vi "Serial Log Driver.vi"(5 "Scanner 2?  (Scanner1)":bool, 7 "Valid Serial #":bool, 11 "error in (no error)":errorcluster, 12 "Write Text":string[](array[string]), 14 "operation":T1) -> (15 "error out":errorcluster)   [LabVIEW 2013]
uses:
  Controls/File Driver States.ctl
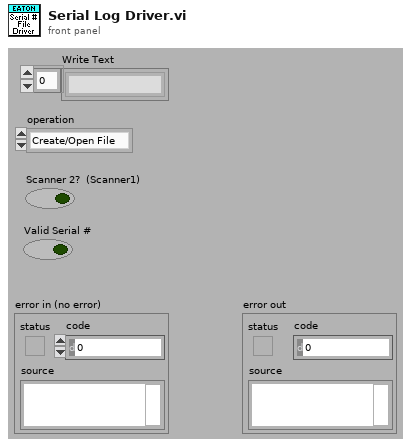
[diagram p1: front panel]
types:
  T1 = typedef "File Driver States.ctl" = enum16{"Create/Open File", "Write File", "Close File"}
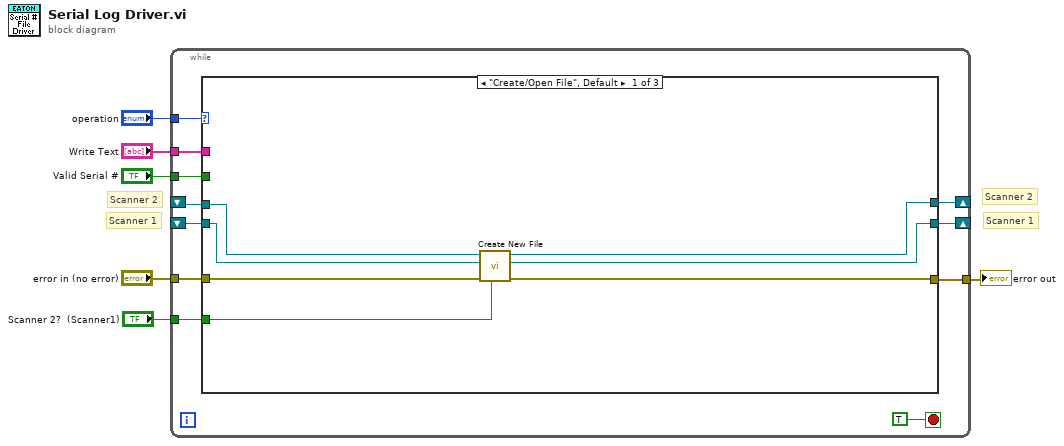
[diagram p0: block diagram]
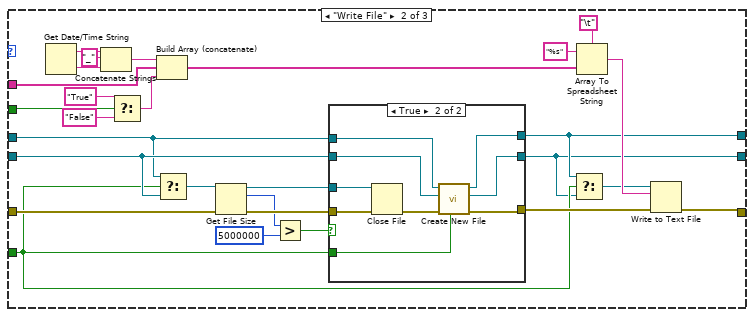
[diagram p2: hidden frame]
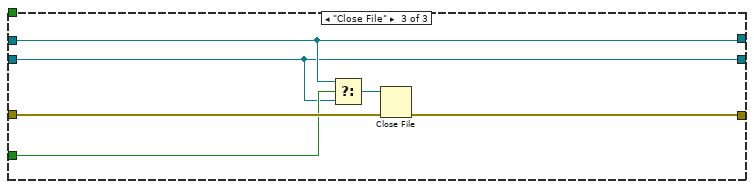
[diagram p4: hidden frame]
diagram:
  # "Scanner 2"
  # "Scanner 1"
  # "Scanner 2"
  # "Scanner 1"
  n1 = while {
    tunnel: "Write Text" -> [w17]
    tunnel: "error in (no error)" -> [w16]
    tunnel: [w15] -> w4
    tunnel: "Scanner 2?  (Scanner1)" -> [w11]
    shift-right: [w12] -> _
    shift-left: _ -> [w13]
    shift-right: [w10] -> _
    shift-left: _ -> [w9]
    tunnel: "operation" -> [w14]
    tunnel: "Valid Serial #" -> [w8]
    stop <- TRUE stop-if-true
    n2 = case shown="\"Create/Open File\", Default" w14 {
      tunnel: w16 -> [w23 w52 w70]
      tunnel: w17 -> [_ w34 _]
      tunnel: [w19 w36 w66] -> w12
      tunnel: [w24 w39 w69] -> w15
      tunnel: w13 -> [w20 w46 w66]
      tunnel: w11 -> [w18 w38 w68]
      tunnel: [w22 w37 w67] -> w10
      tunnel: w9 -> [w21 w44 w67]
      tunnel: w8 -> [_ w28 _]
      frame "Create/Open File", Default {
        n3 = call "Create New File.vi"("Scanner 2?  (Scanner1)"=w18, "error in (no error)"=w23, "Scanner 1"=w20, "Scanner 2"=w21) -> ("error out"=w24:errorcluster, "Scanner 1 File out"=w19:refnum<file>, "Scanner 2 File out"=w22:refnum<file>)  [unwired: 5 in]
      }
      frame "Write File" {
        n4 = Get Date/Time String() -> (date string=w33:string, time string=w32:string)  [unwired: 3 in]
        n5 = Concatenate Strings(w33, "_" ("string"), w32) -> (w30:string)
        n6 = Select(t="True" ("string"), s=w28, f="False") -> (s? t:f=w25:string)
        n7 = Build Array (concatenate)(w30, w34, w25) -> (w29:string[])
        n8 = Select(t=w44, s=w38, f=w46) -> (s? t:f=w50:refnum<file>)
        n9 = Get File Size(file=w50, error in=w52) -> (refnum out=w49:refnum<file>, size (in bytes)=w48:i64, 0:w51:errorcluster)
        n10 = Greater?(x=w48, y=i64 5000000) -> (0:w45:bool)
        n11 = case shown="True" w45 {
          tunnel: [w55 w63] -> w40
          tunnel: w51 -> [w55 w64]
          tunnel: w49 -> [_ w56]
          tunnel: w46 -> [w54 w62]
          tunnel: w44 -> [w53 w61]
          tunnel: w38 -> [_ w60]
          tunnel: [w54 w59] -> w36
          tunnel: [w53 w58] -> w37
          frame False {
          }
          frame True {
            n12 = Close File(refnum=w56, error in=w64) -> (error out=w57:errorcluster)  [unwired: 1 out]
            n13 = call "Create New File.vi"("Scanner 2?  (Scanner1)"=w60, "error in (no error)"=w57, "Scanner 1"=w62, "Scanner 2"=w61) -> ("error out"=w63:errorcluster, "Scanner 1 File out"=w59:refnum<file>, "Scanner 2 File out"=w58:refnum<file>)  [unwired: 5 in]
          }
        }
        n14 = Select(t=w37, s=w38, f=w36) -> (s? t:f=w35:refnum<file>)
        n15 = Array To Spreadsheet String(delimiter (Tab)="\t", array=w29, 3:"%s" ("format string")) -> (spreadsheet string=w43:string)
        n16 = Write to Text File(file (use dialog)=w35, text=w43, error in=w40) -> (error out=w39:errorcluster)  [unwired: 1 in, 2 out]
      }
      frame "Close File" {
        n17 = Select(t=w67, s=w68, f=w66) -> (s? t:f=w65:refnum<file>)
        n18 = Close File(refnum=w65, error in=w70) -> (error out=w69:errorcluster)  [unwired: 1 out]
      }
    }
  }
  "error out" <- w4
